vi "HF modbus (com3).vi"(4 "State":i16, 5 "Time":dbl format="%.2f", 6 "Sensor Values":dbl[](array[numeric]), 7 "Set Points":dbl[](array[numeric])=[1.0]) -> (0 "required data":T1={"Set Point names"=["unitID (usually 1)"], "required number of setpoints"=1, "required number of sensors"=0, "Sensor names"=[]}, 3 "output value":dbl)   [LabVIEW 2019]
panel:
  in  "error in (no error)":errorcluster
  out "UnitID":i32
  out "read buffer":string
  # "Enter the correct information for this control code in the required data structure below. Then make the current value default by right clicking on the border of the data structure. Select \"data operations\" and then select \"make current value default\". These values will be displayed by process controller."
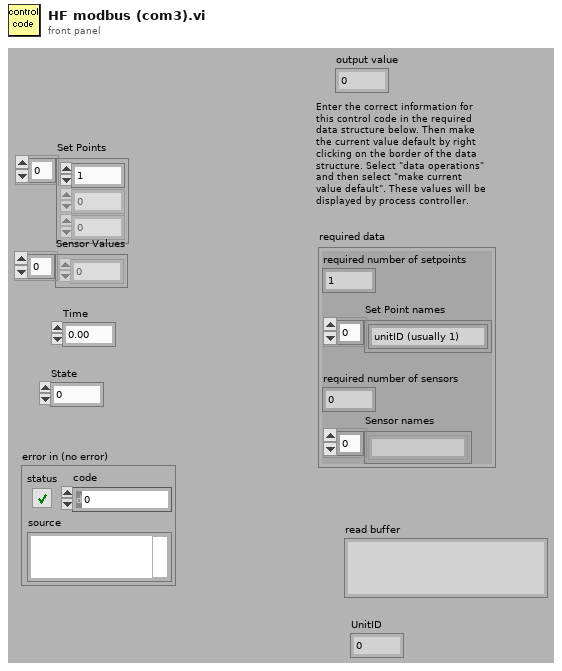
[diagram p1: front panel]
types:
  T1 = cluster{"Set Point names":string[], "required number of setpoints":u8, "required number of sensors":u8, "Sensor names":string[]}
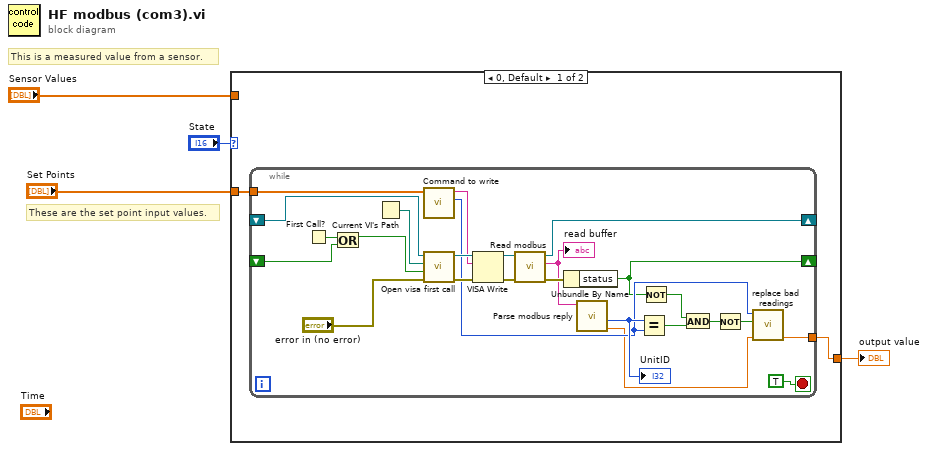
[diagram p0: block diagram]
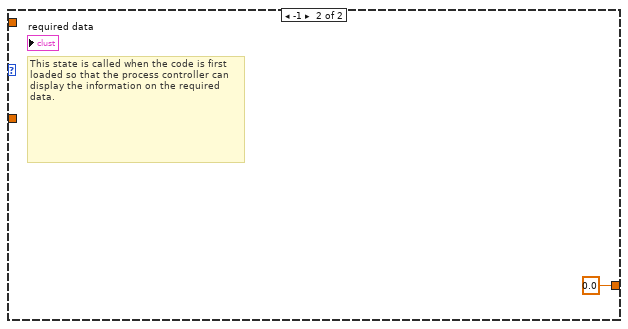
[diagram p2: hidden frame]
diagram:
  # "These are the set point input values."
  # "This is a measured value from a sensor."
  n1 = case shown="0, Default" "State" {
    tunnel: [w6 0.0 ("fraction on")] -> w3
    tunnel: "Set Points" -> [w5 _]
    tunnel: "Sensor Values" -> [_ _]
    frame 0, Default {
      n2 = while {
        tunnel: [w10] -> w6
        shift-right: [w21] -> _
        shift-left: _ -> [w20]
        tunnel: w5 -> [w18]
        shift-right: [w9] -> _
        shift-left: _ -> [w7]
        stop <- TRUE stop-if-true
        n3 = First Call?() -> (First Call?: T/F=w27:bool)
        n4 = Or(x=w27, y=w7) -> (x .or. y?=w8:bool)
        n5 = Current VI's Path() -> (path=w16:path)
        n6 = call "Command to write.vi"("Set Points"=w18) -> ("Unit ID"=w13:i32, "Command to write"=w17:string)  [unwired: 9 in]
        n7 = call "Open visa first call.vi"("error in (no error)"="error in (no error)", "First Call?: T/F"=w8, "Com port"=w16, "VISA Refnum in"=w20) -> ("error out"=w23:errorcluster, "VISA Refnum out"=w30:refnum<visa-resource-name>)  [unwired: 6 in]
        n8 = VISA Write(VISA resource name=w30, write buffer=w17, error in (no error)=w23) -> (VISA resource name out=w29:refnum<visa-resource-name>, error out=w28:errorcluster)  [unwired: 1 out]
        n9 = call "Read modbus.vi"("error in (no error)"=w28, "VISA Refnum in"=w29) -> ("error out"=w19:errorcluster, "read buffer"=w14:string, "VISA Refnum out"=w21:refnum<visa-resource-name>)  [unwired: 7 in]
        "read buffer" <- w14
        n10 = Unbundle By Name(w19) -> ("status"=w9:bool)
        n11 = call "Parse modbus reply.vi"("read buffer"=w14) -> ("Meter reading"=w11:sgl, "UnitID"=w15:i32)  [unwired: 9 in]
        "UnitID" <- w15
        n12 = Equal?(x=w15, y=w13) -> (x = y?=w25:bool)
        n13 = Not(x=w9) -> (.not. x?=w26:bool)
        n14 = And(x=w26, y=w25) -> (x .and. y?=w24:bool)
        n15 = Not(x=w24) -> (.not. x?=w12:bool)
        n16 = call "replace bad readings.vi"("Meter reading in"=w11, "bad data read"=w12, "Unit ID"=w13) -> ("Meter reading out"=w10:dbl)  [unwired: 8 in]
      }
    }
    frame -1 {
      # "This state is called when the code is first loaded so that the process controller can display the information on the required data."
    }
  }
  "output value" <- w3
